vi "Serial ADB WrRd.vi"(4 "Read Delay (ms)":u32=250, 6 "Write Wait (mS)":u16=10, 8 "handle":u32, 9 "Write String":string, 10 "Baud Rate":u32=115200, 11 "Description":string="TTL232RG-3V3_Application") -> (1 "Read Buffer":string)   [LabVIEW 2018]
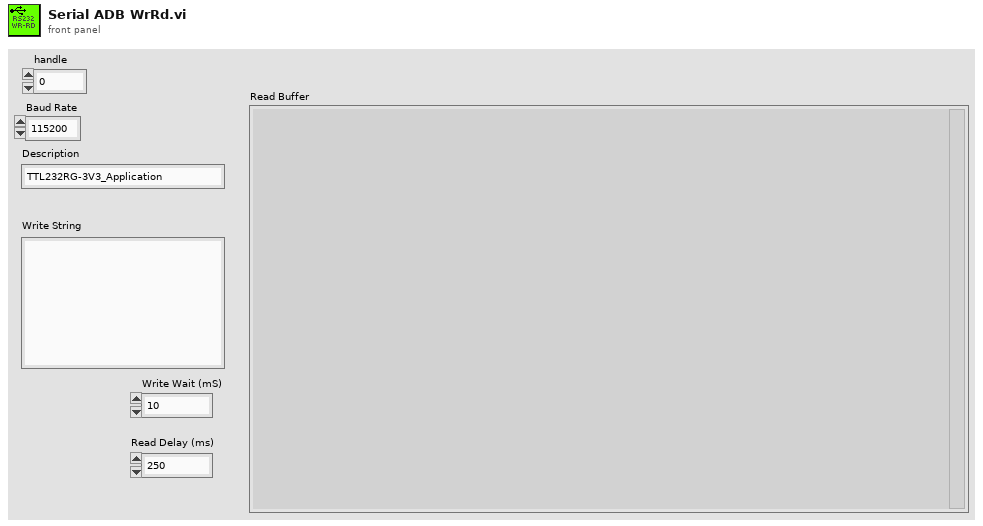
[diagram p1: front panel]
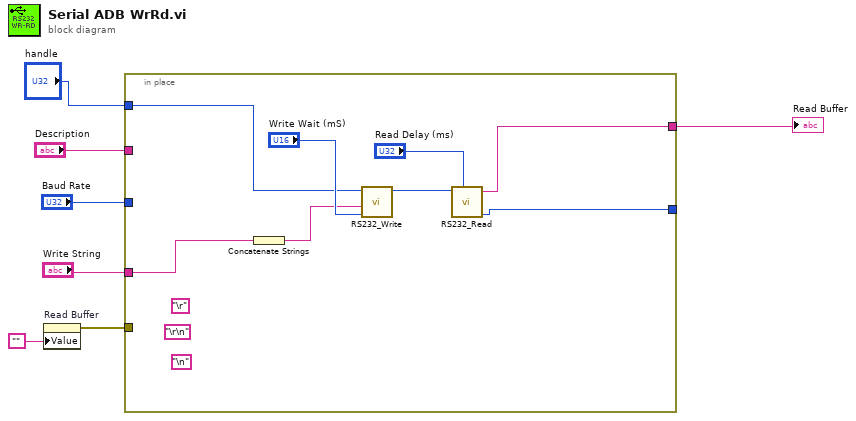
[diagram p0: block diagram]
diagram:
  n1 = property on="Read Buffer" class="Str"("Value"="") -> (error out=w3:errorcluster)  [unwired: 2 in, 1 out]
  n2 = in-place {
    in-place-border: "Description" -> [_]
    in-place-border: "Baud Rate" -> [_]
    in-place-border: "Write String" -> [w9]
    in-place-border: [w12] -> w4
    in-place-border: w3 -> [_]
    in-place-border: "handle" -> [w11]
    in-place-border: [w10] -> _
    (unwired) "\n"
    (unwired) "\r\n"
    (unwired) "\r"
    n3 = Concatenate Strings(w9) -> (w8:string)
    n4 = call "RS232_Write.vi"("Wait (mS)"="Write Wait (mS)", "Write Buffer"=w8, "Handle"=w11) -> ("Handle Out"=w14:u32)  [unwired: 7 in, 1 out]
    n5 = call "RS232_Read.vi"("Read Delay (ms)"="Read Delay (ms)", "Handle"=w14) -> ("Handle Out"=w10:u32, "Read Buffer"=w12:string)  [unwired: 7 in, 1 out]
  }
  "Read Buffer" <- w4
